vi "XML Example.vi"() -> ()   [LabVIEW 2021, in "Tree Map.lvlib"]
doc: "<b>Author:</b> Piotr Kruczkowski <PrimaryKey>\n<b>License:</b> NewBSD\n\nCopyright (c) 2019, National Instruments\nAll rights reserved.\n\nRedistribution and use in source and binary forms, with or without\nmodification, are permitted provided that the following conditions are met:\n1. Redistributions of source code must retain the above copyright\n notice, this list of conditions and the following disclaimer.\n2. Redistributions in binary form must reproduce the above copyright\n notice, this list of conditions and the following disclaimer in the\n documentation and/or other materials provided with the distribution.\n3. Neither the name of National Instruments nor the\n names of its contributors may be used to endorse or promote products\n derived from this software without specific prior written permission.\n\nTHIS SOFTWARE IS PROVIDED BY National Instruments ''AS IS'' AND ANY\nEXPRESS OR IMPLIED WARRANTIES, INCLUDING, BUT NOT LIMITED TO, THE IMPLIED\nWARRANTIES OF MERCHANTABILITY AND FITNESS FOR A PARTICULAR PURPOSE ARE\nDISCLAIMED. IN NO EVENT SHALL National Instruments BE LIABLE FOR ANY\nDIRECT, INDIRECT, INCIDENTAL, SPECIAL, EXEMPLARY, OR CONSEQUENTIAL DAMAGES\n(INCLUDING, BUT NOT LIMITED TO, PROCUREMENT OF SUBSTITUTE GOODS OR SERVICES;\nLOSS OF USE, DATA, OR PROFITS; OR BUSINESS INTERRUPTION) HOWEVER CAUSED AND\nON ANY THEORY OF LIABILITY, WHETHER IN CONTRACT, STRICT LIABILITY, OR TORT\n(INCLUDING NEGLIGENCE OR OTHERWISE) ARISING IN ANY WAY OUT OF THE USE OF THIS\nSOFTWARE, EVEN IF ADVISED OF THE POSSIBILITY OF SUCH DAMAGE."
uses:
  <vilib>/National Instruments/Tree Map/Tree Map.lvlib
panel:
  out "Tree XML After Unflattening":string="<Base>\nThis is the base root.\n    <Info>\n        This is a node with information in it.\n        <Value Attr=\"Foo\" Attr2=\"Bar\">0</Value>\r\n        <Value Attr=\"Foo\" Attr2=\"Bar\">1</Value>\r\n        <Value Attr=\"Foo\" Attr2=\"Bar\">2</Value>\n    </Info>\n</Base>"
  out "Tree XML Pre Flattening":string="<Base>\nThis is the base root.\n    <Info>\n        This is a node with information in it.\n        <Value Attr=\"Foo\" Attr2=\"Bar\">0</Value>\r\n        <Value Attr=\"Foo\" Attr2=\"Bar\">1</Value>\r\n        <Value Attr=\"Foo\" Attr2=\"Bar\">2</Value>\n    </Info>\n</Base>"
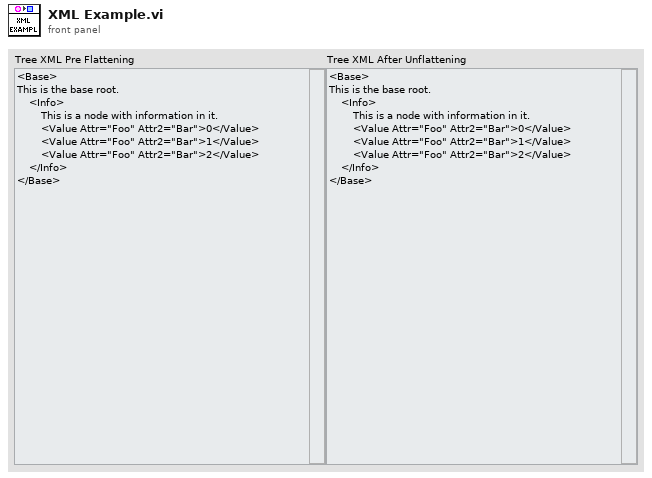
[diagram p1: front panel]
types:
  T1 = typedef "Tree Map.lvlib/Tree Map Data.ctl" = map{string, cluster{"Child Paths Set":set{string}, "Name":string, "Data":string, "Attributes":map{string, string}}}
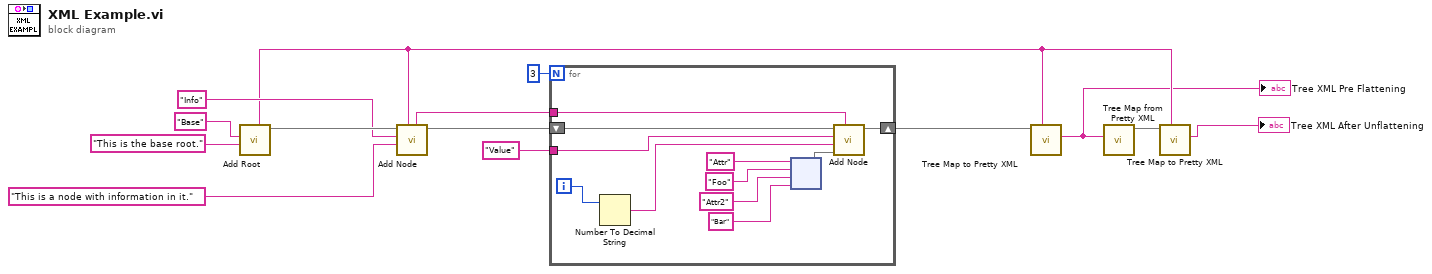
[diagram p0: block diagram]
diagram:
  n1 = call <vilib>:"Add Root.vi"("Root Data"="This is the base root." ("Data"), "New Root Name"="Base") -> ("Tree Map Out"=w13:T1, "Root Path"=w3:string)  [unwired: 8 in]
  n2 = call <vilib>:"Add Node.vi"("Parent Path"=w3, "Data"="This is a node with information in it.", "New Node Name"="Info" ("New Branch Name"), "Tree Map In"=w13) -> ("Tree Map Out"=w12:T1, "New Node Path"=w9:string)  [unwired: 5 in, 1 out]
  n3 = for {
    N: 3 -> [_]
    shift-right: [w21] -> w4
    shift-left: w12 -> [w25]
    tunnel: w9 -> [w23]
    tunnel: "Value" ("format string") -> [w15]
    i -> [w24]
    n4 = Number To Decimal String(number=w24) -> (decimal integer string=w22:string)  [unwired: 1 in]
    n5 = node("Attr" ("key"), "Foo" ("key"), "Attr2" ("key"), "Bar" ("key")) -> (w18:map{string, string})
    n6 = call <vilib>:"Add Node.vi"("Parent Path"=w23, "Attributes"=w18, "Data"=w22, "New Node Name"=w15, "Tree Map In"=w25) -> ("Tree Map Out"=w21:T1)  [unwired: 4 in, 2 out]
  }
  n7 = call <vilib>:"Tree Map to Pretty XML.vi"("Root Path"=w3, "Tree Map In"=w4) -> ("Pretty XML"=w2:string)  [unwired: 8 in, 1 out]
  "Tree XML Pre Flattening" <- w2
  n8 = call <vilib>:"Tree Map from Pretty XML.vi"("Pretty XML"=w2) -> ("Tree Map Out"=w5:T1)  [unwired: 9 in, 1 out]
  n9 = call <vilib>:"Tree Map to Pretty XML.vi"("Root Path"=w3, "Tree Map In"=w5) -> ("Pretty XML"=→"Tree XML After Unflattening":string)  [unwired: 8 in, 1 out]
